vi "Add Minor Frame.vi"(7 "minorFramePeriod":i32, 8 "error in":errorcluster, 9 "messageRefs":string[](array[string]), 10 "name":string, 11 "channel in":refnum<k24>) -> (0 "error out":errorcluster, 2 "new minor frame":refnum<k24>, 3 "channel out":refnum<k24>)   [LabVIEW 2020, in "AIM_1553_Parameter_ni.lvlib"]
uses:
  AIM_1553_Parameter_ni.lvlib
  C:/Users/Administrator/Desktop/GIT/Ballard-Arinc-429-XML-Generator/Source/Assemblies/Aim_1553_Parameter_ni/bin/Debug/AIM_1553_Parameter_ni.dll
  Assemblies/Aim_1553_Parameter_ni/bin/Debug/AIM_1553_Parameter_ni.dll
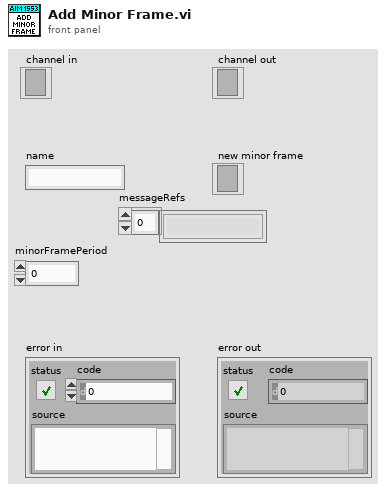
[diagram p1: front panel]
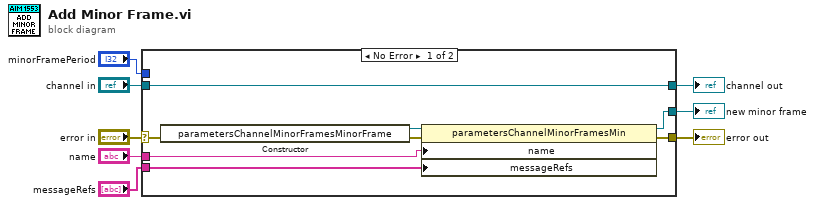
[diagram p0: block diagram]
diagram:
  n1 = case shown="No Error" "error in" {
    selector: "error in" -> [w9 w17]
    tunnel: [w10 w18] -> w8
    tunnel: [w14 w17] -> w7
    tunnel: "channel in" -> [w10 w18]
    tunnel: [w13 _] -> w4
    tunnel: "name" -> [w12 _]
    tunnel: "minorFramePeriod" -> [_ _]
    tunnel: "messageRefs" -> [w11 _]
    frame No Error {
      n2 = constructor class="parametersChannelMinorFramesMin"(error in=w9) -> (reference out=w15:refnum<k24>, error out=w16:errorcluster)  [unwired: 2 in, 1 out]
      n3 = property class="parametersChannelMinorFramesMin"(reference=w15, error in=w16, "name"=w12, "messageRefs"=w11) -> (reference out=w13:refnum<k24>, error out=w14:errorcluster)
    }
    frame Error {
    }
  }
  "channel out" <- w8
  "error out" <- w7
  "new minor frame" <- w4
